vi "VI Tree.vi"   [LabVIEW 2018, in "LTB-1.lvlib" / "3150.lvlib"]
doc: "This is the instrument driver for the EXFO 3150 module. The VI Tree displays all the user-callable VIs of the instrument driver in an organized table."
uses:
  3150.lvlib
panel:
  # "(c) 2010 EXFO Inc. ALL RIGHTS RESERVED."
  # "SEE DIAGRAM\nFOR VI TREE."
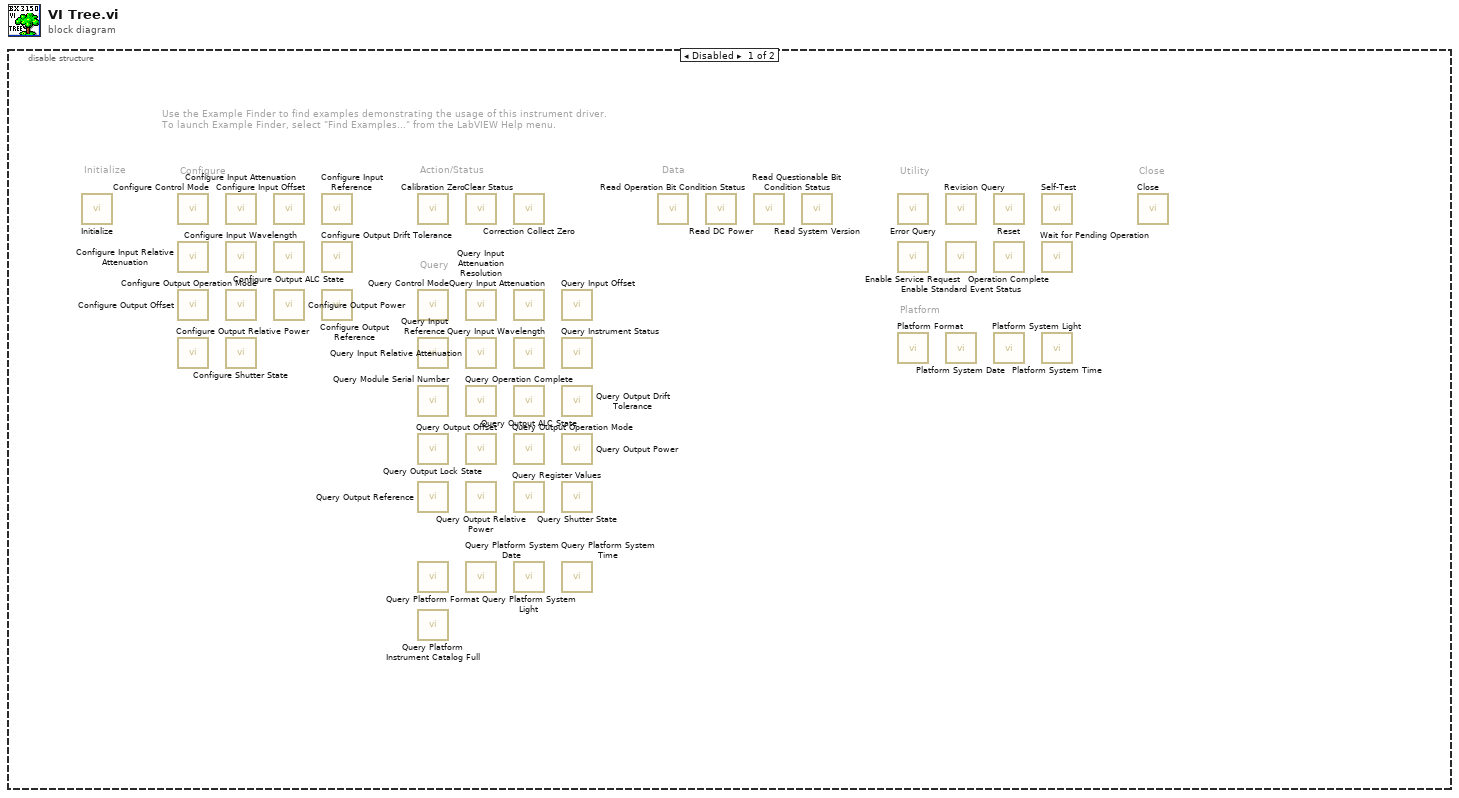
[diagram p0: block diagram]
diagram:
  n1 = disable-structure shown="Disabled" {
    frame Disabled {
      # "Query"
      # "Platform"
      # "Utility"
      # "Data"
      # "Use the Example Finder to find examples demonstrating the usage of this instrument driver.\nTo launch Example Finder, select \"Find Examples...\" from the LabVIEW Help menu."
      # "Configure"
      # "Action/Status"
      # "Close"
      # "Initialize"
      n2 = call "Initialize.vi"() -> ()  [unwired: 10 in, 2 out]
      n3 = call "Configure Control Mode.vi"() -> ()  [unwired: 10 in, 2 out]
      n4 = call "Configure Input Relative Attenuation.vi"() -> ()  [unwired: 14 in, 2 out]
      n5 = call "Configure Output Offset.vi"() -> ()  [unwired: 14 in, 2 out]
      n6 = call "Configure Output Relative Power.vi"() -> ()  [unwired: 14 in, 2 out]
      n7 = call "Configure Input Attenuation.vi"() -> ()  [unwired: 14 in, 2 out]
      n8 = call "Configure Input Wavelength.vi"() -> ()  [unwired: 14 in, 2 out]
      n9 = call "Configure Output Operation Mode.vi"() -> ()  [unwired: 10 in, 2 out]
      n10 = call "Configure Shutter State.vi"() -> ()  [unwired: 10 in, 2 out]
      n11 = call "Configure Input Offset.vi"() -> ()  [unwired: 14 in, 2 out]
      n12 = call "Configure Output ALC State.vi"() -> ()  [unwired: 10 in, 2 out]
      n13 = call "Configure Output Power.vi"() -> ()  [unwired: 14 in, 2 out]
      n14 = call "Configure Input Reference.vi"() -> ()  [unwired: 14 in, 2 out]
      n15 = call "Configure Output Drift Tolerance.vi"() -> ()  [unwired: 14 in, 2 out]
      n16 = call "Configure Output Reference.vi"() -> ()  [unwired: 14 in, 2 out]
      n17 = call "Calibration Zero.vi"() -> ()  [unwired: 10 in, 2 out]
      n18 = call "Query Control Mode.vi"() -> ()  [unwired: 9 in, 3 out]
      n19 = call "Query Input Reference.vi"() -> ()  [unwired: 9 in, 3 out]
      n20 = call "Query Module Serial Number.vi"() -> ()  [unwired: 9 in, 3 out]
      n21 = call "Query Output Lock State.vi"() -> ()  [unwired: 9 in, 3 out]
      n22 = call "Query Output Reference.vi"() -> ()  [unwired: 9 in, 3 out]
      n23 = call "Query Platform Format.vi"() -> ()  [unwired: 8 in, 4 out]
      n24 = call "Query Platform Instrument Catalog Full.vi"() -> ()  [unwired: 9 in, 3 out]
      n25 = call "Clear Status.vi"() -> ()  [unwired: 14 in, 2 out]
      n26 = call "Query Input Attenuation Resolution.vi"() -> ()  [unwired: 9 in, 3 out]
      n27 = call "Query Input Relative Attenuation.vi"() -> ()  [unwired: 9 in, 3 out]
      n28 = call "Query Operation Complete.vi"() -> ()  [unwired: 9 in, 3 out]
      n29 = call "Query Output Offset.vi"() -> ()  [unwired: 9 in, 3 out]
      n30 = call "Query Output Relative Power.vi"() -> ()  [unwired: 9 in, 3 out]
      n31 = call "Query Platform System Date.vi"() -> ()  [unwired: 11 in, 5 out]
      n32 = call "Correction Collect Zero.vi"() -> ()  [unwired: 10 in, 2 out]
      n33 = call "Query Input Attenuation.vi"() -> ()  [unwired: 9 in, 3 out]
      n34 = call "Query Input Wavelength.vi"() -> ()  [unwired: 9 in, 3 out]
      n35 = call "Query Output ALC State.vi"() -> ()  [unwired: 9 in, 3 out]
      n36 = call "Query Output Operation Mode.vi"() -> ()  [unwired: 9 in, 3 out]
      n37 = call "Query Register Values.vi"() -> ()  [unwired: 9 in, 3 out]
      n38 = call "Query Platform System Light.vi"() -> ()  [unwired: 9 in, 3 out]
      n39 = call "Query Input Offset.vi"() -> ()  [unwired: 9 in, 3 out]
      n40 = call "Query Instrument Status.vi"() -> ()  [unwired: 9 in, 3 out]
      n41 = call "Query Output Drift Tolerance.vi"() -> ()  [unwired: 9 in, 3 out]
      n42 = call "Query Output Power.vi"() -> ()  [unwired: 9 in, 3 out]
      n43 = call "Query Shutter State.vi"() -> ()  [unwired: 9 in, 3 out]
      n44 = call "Query Platform System Time.vi"() -> ()  [unwired: 11 in, 5 out]
      n45 = call "Read Operation Bit Condition Status.vi"() -> ()  [unwired: 9 in, 3 out]
      n46 = call "Read DC Power.vi"() -> ()  [unwired: 9 in, 3 out]
      n47 = call "Read Questionable Bit Condition Status.vi"() -> ()  [unwired: 9 in, 3 out]
      n48 = call "Read System Version.vi"() -> ()  [unwired: 9 in, 3 out]
      n49 = call "Error Query.vi"() -> ()  [unwired: 8 in, 4 out]
      n50 = call "Enable Service Request.vi"() -> ()  [unwired: 10 in, 2 out]
      n51 = call "Platform Format.vi"() -> ()  [unwired: 10 in, 2 out]
      n52 = call "Revision Query.vi"() -> ()  [unwired: 8 in, 4 out]
      n53 = call "Enable Standard Event Status.vi"() -> ()  [unwired: 10 in, 2 out]
      n54 = call "Platform System Date.vi"() -> ()  [unwired: 10 in, 2 out]
      n55 = call "Reset.vi"() -> ()  [unwired: 10 in, 2 out]
      n56 = call "Operation Complete.vi"() -> ()  [unwired: 10 in, 2 out]
      n57 = call "Platform System Light.vi"() -> ()  [unwired: 10 in, 2 out]
      n58 = call "Self-Test.vi"() -> ()  [unwired: 9 in, 3 out]
      n59 = call "Wait for Pending Operation.vi"() -> ()  [unwired: 10 in, 2 out]
      n60 = call "Platform System Time.vi"() -> ()  [unwired: 10 in, 2 out]
      n61 = call "Close.vi"() -> ()  [unwired: 11 in, 1 out]
    }
    frame Enabled {
    }
  }
